vi "TestDLLWrapper.vi"(2 "error in (no error)":errorcluster, 3 "Input":T2) -> (0 "error out":errorcluster, 1 "Output":T1)   [LabVIEW 2023]
uses:
  DLL-RRT/x64/RRT.dll
  RRTOutput.ctl
  RRTInput.ctl
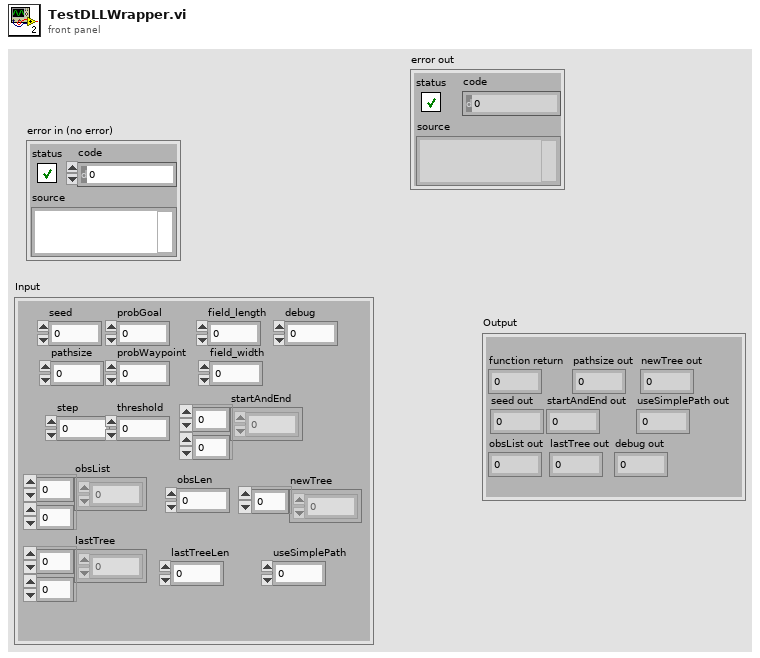
[diagram p1: front panel]
types:
  T1 = typedef "RRTOutput.ctl" = cluster{"function return":i32, "seed out":i32, "pathsize out":i32, "startAndEnd out":sgl, "obsList out":sgl, "lastTree out":sgl, "newTree out":sgl, "useSimplePath out":i32, "debug out":sgl}
  T2 = typedef "RRTInput.ctl" = cluster{"seed":i32, "pathsize":i32, "probGoal":sgl, "probWaypoint":sgl, "step":sgl, "threshold":sgl, "field_length":sgl, "field_width":sgl, "startAndEnd":sgl[][], "obsList":sgl[][], "obsLen":i32, "lastTree":sgl[][], "lastTreeLen":i32, "newTree":sgl[], "useSimplePath":i32, "debug":sgl}
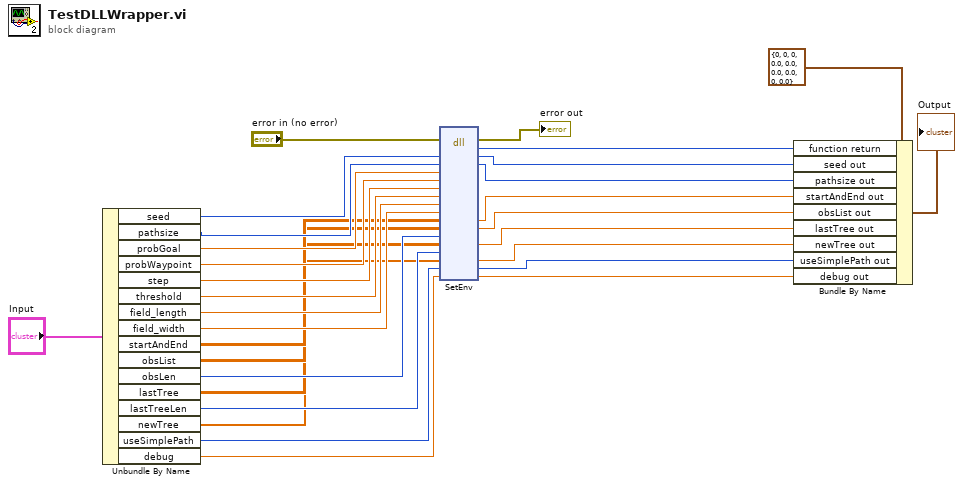
[diagram p0: block diagram]
diagram:
  n1 = Unbundle By Name("Input") -> ("seed"=w25:i32, "pathsize"=w24:i32, "probGoal"=w23:sgl, "probWaypoint"=w22:sgl, "step"=w21:sgl, "threshold"=w20:sgl, "field_length"=w19:sgl, "field_width"=w18:sgl, "startAndEnd"=w17:sgl[][], "obsList"=w16:sgl[][], "obsLen"=w15:i32, "lastTree"=w14:sgl[][], "lastTreeLen"=w13:i32, "newTree"=w12:sgl[], "useSimplePath"=w11:i32, "debug"=w10:sgl)
  n2 = dll-call lib="C:/Users/ebert/Documents/codes/SSL/repo/SSL_AI/DLL-RRT/x64/RRT.*" fn="SetEnv"(error in="error in (no error)", "seed"=w25, "pathsize"=w24, "probGoal"=w23, "probWaypoint"=w22, "step"=w21, "threshold"=w20, "field_length"=w19, "field_width"=w18, "startAndEnd"=w17, "obsList"=w16, "obsLen"=w15, "lastTree"=w14, "lastTreeLen"=w13, "newTree"=w12, "useSimplePath"=w11, "debug"=w10) -> (error out=→"error out":errorcluster, w9:i32, "seed"=w8:i32, "pathsize"=w7:i32, "startAndEnd"=w6:sgl, "obsList"=w5:sgl, "lastTree"=w4:sgl, "newTree"=w3:sgl, "useSimplePath"=w2:i32, "debug"=w1:sgl)  [unwired: 10 in, 1 out]
  n3 = Bundle By Name(cluster=T1 {"function return"=0, "seed out"=0, "pathsize out"=0, "startAndEnd out"=0.0, "obsList out"=0.0, "lastTree out"=0.0, "newTree out"=0.0, "useSimplePath out"=0, "debug out"=0.0} ("Output"), "function return"=w9, "seed out"=w8, "pathsize out"=w7, "startAndEnd out"=w6, "obsList out"=w5, "lastTree out"=w4, "newTree out"=w3, "useSimplePath out"=w2, "debug out"=w1) -> (→"Output":T1)
